vi "Helium4 Temperature 2 Pressure.vi"(11 "He4 Temperature (K)":dbl=0.4 format="%_6f") -> (3 "He4 Pressure (mbar)":dbl format="%#_5e")   [LabVIEW 2020]
uses:
  <vilib>/Analysis/polynomials.llb/Scalar Polynomial Evaluation (DBL).vi
  <vilib>/Analysis/NI_AALPro.lvlib
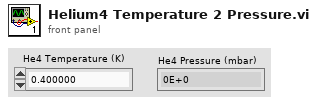
[diagram p1: front panel]
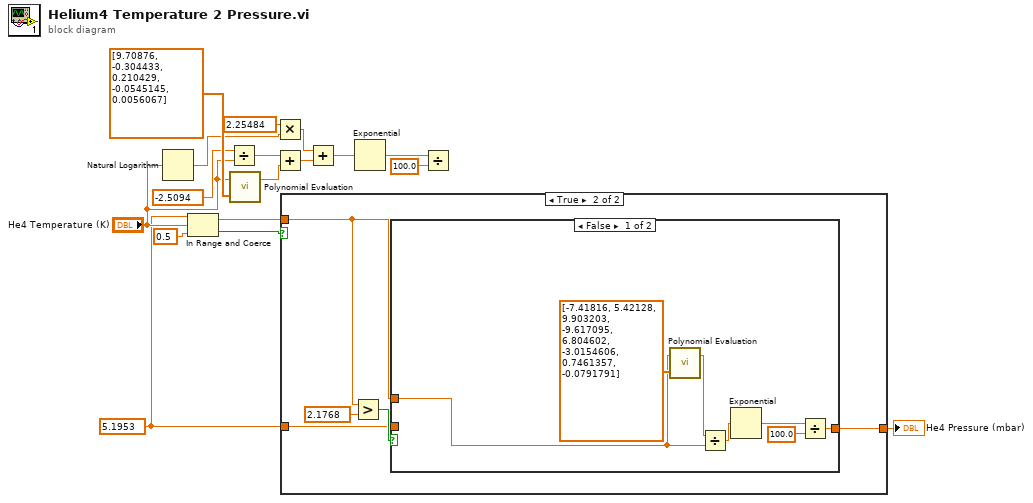
[diagram p0: block diagram]
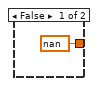
[diagram p2: hidden frame]
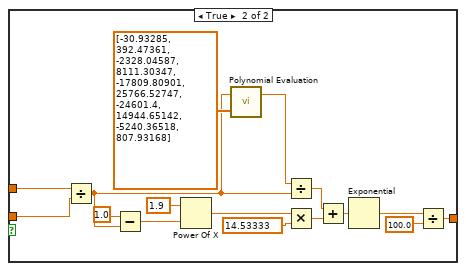
[diagram p3: hidden frame]
diagram:
  w2 = 5.1953 ("upper limit")
  n1 = Natural Logarithm(1:"He4 Temperature (K)") -> (0:w13:dbl)
  n2 = In Range and Coerce(upper limit=w2, x="He4 Temperature (K)", lower limit=0.5) -> (coerced(x)=w3:dbl, In Range?=w4:bool)
  n3 = Divide(x=-2.5094, y="He4 Temperature (K)") -> (x/y=w15:dbl)
  n4 = call-poly <vilib>:"Polynomial Evaluation.vi"("P(x)"=dbl[] [9.70876, -0.304433, 0.210429, -0.0545145, 0.0056067], "a"="He4 Temperature (K)") -> ("P(a)"=w14:dbl)  [unwired: 1 out]
  n5 = Multiply(x=2.25484 ("y"), y=w13) -> (x*y=w11:dbl)
  n6 = Add(x=w15, y=w14) -> (x+y=w10:dbl)
  n7 = case shown="True" w4 {
    tunnel: [nan ("y") w19] -> w1
    tunnel: w3 -> [_ w21]
    tunnel: w2 -> [_ w20]
    frame False {
    }
    frame True {
      n8 = Greater?(x=w21, y=2.1768) -> (0:w22:bool)
      n9 = case shown="False" w22 {
        tunnel: w21 -> [w28 w44]
        tunnel: w20 -> [_ w46]
        tunnel: [w25 w31] -> w19
        frame False {
          n10 = call-poly <vilib>:"Polynomial Evaluation.vi"("P(x)"=dbl[] [-7.41816, 5.42128, 9.903203, -9.617095, 6.804602, -3.0154606, 0.7461357, -0.0791791], "a"=w28) -> ("P(a)"=w29:dbl)  [unwired: 1 out]
          n11 = Divide(x=w29, y=w28) -> (x/y=w27:dbl)
          n12 = Exponential(1:w27) -> (0:w24:dbl)
          n13 = Divide(x=w24, y=100.0) -> (x/y=w25:dbl)
        }
        frame True {
          n14 = Divide(x=w44, y=w46) -> (x/y=w41:dbl)
          n15 = Subtract(x=1.0, y=w41) -> (x-y=w39:dbl)
          n16 = Power Of X(1:w39, 2:1.9 ("y")) -> (0:w37:dbl)
          n17 = call-poly <vilib>:"Polynomial Evaluation.vi"("P(x)"=dbl[] [-30.93285, 392.47361, -2328.04587, 8111.30347, -17809.80901, 25766.52747, -24601.4, 14944.65142, -5240.36518, 807.93168], "a"=w41) -> ("P(a)"=w43:dbl)  [unwired: 1 out]
          n18 = Divide(x=w43, y=w41) -> (x/y=w42:dbl)
          n19 = Multiply(x=w37, y=14.53333) -> (x*y=w35:dbl)
          n20 = Add(x=w42, y=w35) -> (x+y=w34:dbl)
          n21 = Exponential(1:w34) -> (0:w33:dbl)
          n22 = Divide(x=w33, y=100.0) -> (x/y=w31:dbl)
        }
      }
    }
  }
  "He4 Pressure (mbar)" <- w1
  n23 = Add(x=w11, y=w10) -> (x+y=w9:dbl)
  n24 = Exponential(1:w9) -> (0:w8:dbl)
  n25 = Divide(x=w8, y=100.0) -> ()  [unwired: 1 out]
